vi "FlatToRichcif_plugincore_Empty.vi"(5 "OutputClusterType":T1, 11 "InputCluster":T2) -> (3 "OutputCluster":T1)   [LabVIEW 2021, in "CIF_Plugin_Core_server.lvlib"]
uses:
  cif_plugincore_Empty_Flat.ctl
  cif_plugincore_Empty.ctl
  CIF_Plugin_Core_server.lvlib
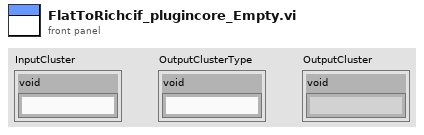
[diagram p1: front panel]
types:
  T1 = typedef "CIF_Plugin_Core_server.lvlib/cif_plugincore_Empty.ctl" = cluster{"void":string}
  T2 = typedef "CIF_Plugin_Core_server.lvlib/cif_plugincore_Empty_Flat.ctl" = cluster{"void":string}
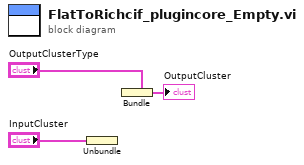
[diagram p0: block diagram]
diagram:
  n1 = Unbundle "Unbundle"("InputCluster") -> ()  [unwired: 1 out]
  n2 = Bundle "Bundle"(cluster="OutputClusterType") -> (→"OutputCluster":T1)  [unwired: 1 in]
